vi "New Task Request.vi"(8 "error in (no error)":errorcluster, 10 "Task":variant, 11 "BuildWorker in":refnum<class "BuildWorker.lvclass">) -> (0 "error out":errorcluster, 3 "BuildWorker out":refnum<class "BuildWorker.lvclass">)   [LabVIEW 2017, in "BuildWorker.lvlib" / "BuildWorker.lvclass"]
uses:
  BuildWorker.lvclass
  Classes/Task Interface/Task/Task.lvclass
  BuildWorker.lvclass/BuildWorker.ctl
  Classes/Task Interface/Task/Status.ctl
  Classes/Task Interface/Task/Task.lvclass/Task.ctl
  Classes/Task Interface/Task/Get Name.vi
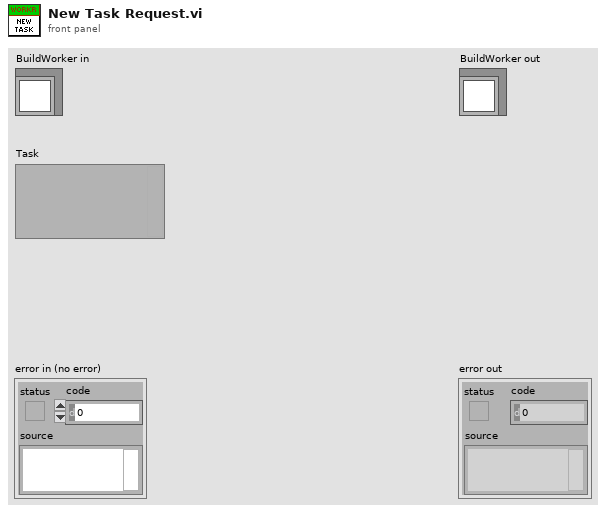
[diagram p1: front panel]
types:
  T1 = typedef "Task Interface.lvlib/Task.lvclass/Status.ctl" = enum16{"Created", "Added", "Pending", "Queued", "Processing", "Cleaning", "Building", "Finished", "Failed", "Removed", "Not found"}
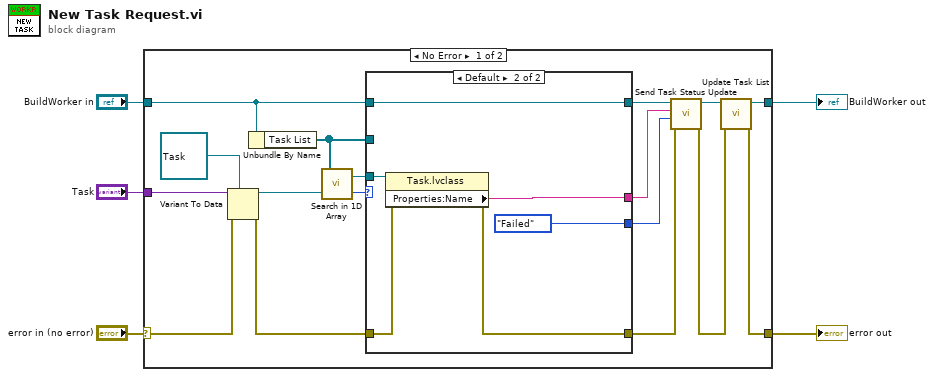
[diagram p0: block diagram]
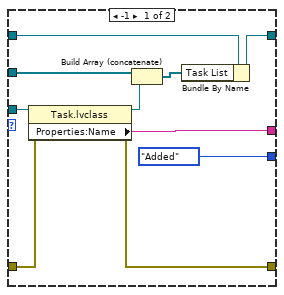
[diagram p2: hidden frame]
diagram:
  n1 = case shown="No Error" "error in (no error)" {
    selector: "error in (no error)" -> [w21 w40]
    tunnel: [w17 w40] -> w4
    tunnel: [w18 w39] -> w2
    tunnel: "BuildWorker in" -> [w20 w39]
    tunnel: "Task" -> [w22 _]
    frame No Error {
      n2 = Variant To Data(error in=w21, type=refnum<class "Task.lvclass"> refnum ("Task Interface.lvlib:Task.lvclass"), Variant=w22) -> (data=w8:refnum<class "Task.lvclass">, error out=w19:errorcluster)
      n3 = Unbundle By Name(w20) -> ("Task List"=w9:refnum<class "Task.lvclass">[])
      n4 = call "Search in 1D Array.vi"("Task in"=w8, "Task Array"=w9) -> ("index of element"=w6:i32, "Task"=w7:refnum<class "Task.lvclass">)
      n5 = case shown="Default" w6 {
        tunnel: w20 -> [w32 w38]
        tunnel: w19 -> [w29 w35]
        tunnel: [w28 w38] -> w16
        tunnel: [w27 w34] -> w14
        tunnel: [w26 w36] -> w12
        tunnel: [Status."Added" ("Status") Status."Failed" ("Status")] -> w11
        tunnel: w9 -> [w25 _]
        tunnel: w7 -> [w24 w37]
        frame -1 {
          n6 = property class="Task.lvclass"(reference=w24, error in=w29) -> (reference out=w30:refnum<class "Task.lvclass">, error out=w27:errorcluster, "Properties:Name"=w26:string)
          n7 = Build Array (concatenate)(w25, w30) -> (w31:refnum<class "Task.lvclass">[])
          n8 = Bundle By Name(cluster=w32, "Task List"=w31) -> (w28:refnum<class "BuildWorker.lvclass">)
        }
        frame Default {
          n9 = property class="Task.lvclass"(reference=w37, error in=w35) -> (error out=w34:errorcluster, "Properties:Name"=w36:string)  [unwired: 1 out]
        }
      }
      n10 = call "Send Task Status Update.vi"("error in (no error)"=w14, "Status"=w11, "Task Name"=w12, "BuildWorker in"=w16) -> ("error out"=w13:errorcluster, "BuildWorker out"=w15:refnum<class "BuildWorker.lvclass">)  [unwired: 6 in]
      n11 = call "Update Task List.vi"("error in (no error)"=w13, "BuildWorker in"=w15) -> ("error out"=w17:errorcluster, "BuildWorker out"=w18:refnum<class "BuildWorker.lvclass">)  [unwired: 8 in]
    }
    frame Error {
    }
  }
  "error out" <- w4
  "BuildWorker out" <- w2
